vi "New coreConfiguration.vi"(6 "core builtInTest configuration (default)":T2, 7 "core sequentialLog configuration (default)":T3={"perChannelStreaming (T)"=TRUE, "useDMA (T)"=TRUE}, 8 "error in":errorcluster, 9 "core timing configuration (default)":T4={"driftMax"=425000000, "delayComp"=0, "irigControlVal"=[0, 0, 0, 0], "irigYears"=2000, "irigType"=1, "jumpThreshPPT"=425000000, "jumpThreshNS"=200000, "timerRollover"=0, "timeSourceSelect"=0, "timeSyncSelect"=0, "timeEnableUserInputThresh"=FALSE, "timeInputThreshVal"=[0, 0], "driftSyncSelect"=0, "driftEnableUserInputThresh"=FALSE, "driftInputThreshVal"=[0, 0], "resolution"=0, "timerValue"=0} {"resolution" items=["Item1NS", "Item1US"]; "driftSyncSelect" items=["None", "PPS0", "PPS1", "PWMIRIG0", "PWMIRIG1", "AMIRIG", "Item10MHZ", "HOST"]; "timeSyncSelect" items=["None", "PPS0", "PPS1", "PWMIRIG0", "PWMIRIG1", "AMIRIG"]; "timeSourceSelect" items=["None", "PPS0", "PPS1", "PWMIRIG0", "PWMIRIG1", "AMIRIG", "Item10MHZ"]; "irigType" items=["A", "B"]}, 10 "core generic configuration (default)":T1) -> (0 "error out":errorcluster, 3 "new CoreConfigurationType":refnum<k24>)   [LabVIEW 2020, in "Ballard_1553_Hardware_ni.lvlib"]
uses:
  Ballard_1553_Hardware_ni.lvlib
  C:/Users/Administrator/Desktop/GIT/Ballard-MIL-STD-1553-Custom-Device/Source/System Explorer/SubVIs/Parse XML Ballard/1.2/BTIXML_SerDes.dll
  Ballard-MIL-STD-1553-Custom-Device/Source/System Explorer/SubVIs/Parse XML Ballard/1.2/BTIXML_SerDes.dll
  _typedefs/core_timing_type.ctl
  _typedefs/core_sequentialLog_type.ctl
  _typedefs/core_builtInTests_type.ctl
  _typedefs/core_generic_type.ctl
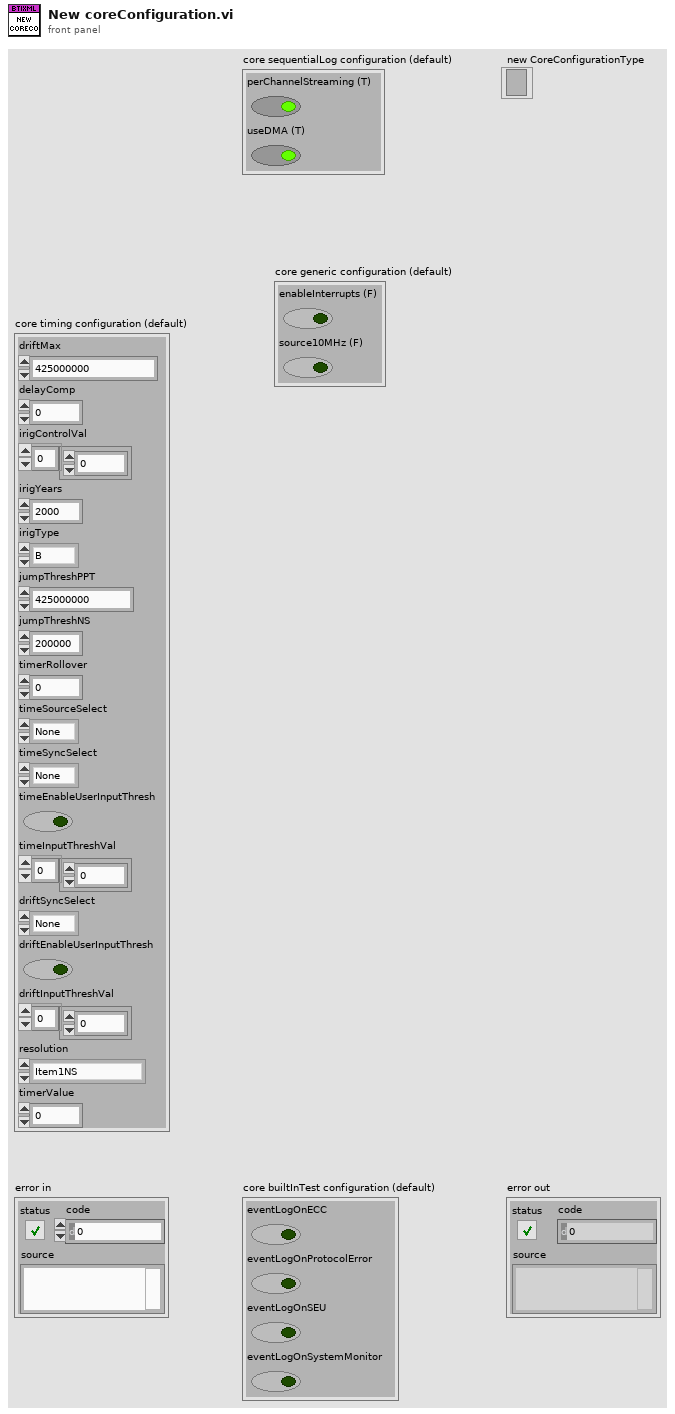
[diagram p1: front panel]
types:
  T1 = typedef "Ballard_1553_Hardware_ni.lvlib/core_generic_type.ctl" = cluster{"enableInterrupts (F)":bool, "source10MHz (F)":bool}
  T2 = typedef "Ballard_1553_Hardware_ni.lvlib/core_builtInTests_type.ctl" = cluster{"eventLogOnECC":bool, "eventLogOnProtocolError":bool, "eventLogOnSEU":bool, "eventLogOnSystemMonitor":bool}
  T3 = typedef "Ballard_1553_Hardware_ni.lvlib/core_sequentialLog_type.ctl" = cluster{"perChannelStreaming (T)":bool, "useDMA (T)":bool}
  T4 = typedef "Ballard_1553_Hardware_ni.lvlib/core_timing_type.ctl" = cluster{"driftMax":u32, "delayComp":i32, "irigControlVal":u8[], "irigYears":u32, "irigType":i32, "jumpThreshPPT":u32, "jumpThreshNS":u32, "timerRollover":u64, "timeSourceSelect":i32, "timeSyncSelect":i32, "timeEnableUserInputThresh":bool, "timeInputThreshVal":u8[], "driftSyncSelect":i32, "driftEnableUserInputThresh":bool, "driftInputThreshVal":u8[], "resolution":i32, "timerValue":u64}
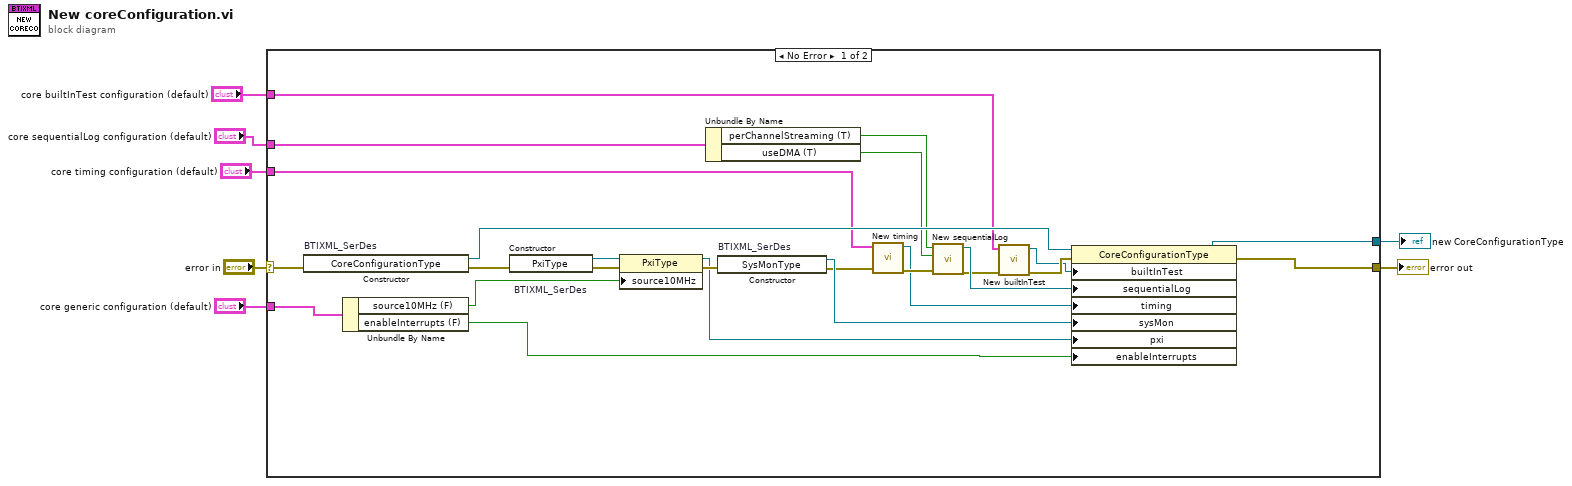
[diagram p0: block diagram]
diagram:
  n1 = case shown="No Error" "error in" {
    selector: "error in" -> [w32 w33]
    tunnel: [w31 w33] -> w6
    tunnel: [w30 _] -> w5
    tunnel: "core timing configuration (default)" -> [w20 _]
    tunnel: "core sequentialLog configuration (default)" -> [w17 _]
    tunnel: "core builtInTest configuration (default)" -> [w11 _]
    tunnel: "core generic configuration (default)" -> [w10 _]
    frame No Error {
      n2 = constructor on="BTIXML_SerDes" class="CoreConfigurationType"(error in=w32) -> (reference out=w23:refnum<k24>, error out=w27:errorcluster)  [unwired: 2 in, 1 out]
      n3 = Unbundle By Name(w10) -> ("source10MHz (F)"=w9:bool, "enableInterrupts (F)"=w8:bool)
      n4 = constructor on="BTIXML_SerDes" class="PxiType"(error in=w27) -> (reference out=w29:refnum<k24>, error out=w28:errorcluster)  [unwired: 2 in, 1 out]
      n5 = property class="PxiType"(reference=w29, error in=w28, "source10MHz"=w9) -> (reference out=w25:refnum<k24>, error out=w26:errorcluster)
      n6 = Unbundle By Name(w17) -> ("perChannelStreaming (T)"=w16:bool, "useDMA (T)"=w15:bool)
      n7 = constructor on="BTIXML_SerDes" class="SysMonType"(error in=w26) -> (reference out=w24:refnum<k24>, error out=w22:errorcluster)  [unwired: 2 in, 1 out]
      n8 = call "New timing.vi"("error in"=w22, "core timeing configuration (default)"=w20) -> ("error out"=w21:errorcluster, "new timing out"=w18:refnum<k24>)  [unwired: 8 in]
      n9 = call "New sequentialLog.vi"("error in"=w21, "useDMA (T)"=w15, "perChannelStreaming (T)"=w16) -> ("error out"=w12:errorcluster, "new sequentialLog out"=w19:refnum<k24>)  [unwired: 7 in]
      n10 = call "New builtInTest.vi"("error in"=w12, "core builtInTest configuration (default)"=w11) -> ("error out"=w14:errorcluster, "new builtInTest out"=w13:refnum<k24>)  [unwired: 8 in]
      n11 = property class="CoreConfigurationType"(reference=w23, error in=w14, "builtInTest"=w13, "sequentialLog"=w19, "timing"=w18, "sysMon"=w24, "pxi"=w25, "enableInterrupts"=w8) -> (reference out=w30:refnum<k24>, error out=w31:errorcluster)
    }
    frame Error {
    }
  }
  "error out" <- w6
  "new CoreConfigurationType" <- w5
